vi "Get Element Write Position.vi"(8 "error in (no error)":errorcluster, 11 "CIPC Reference":u64) -> (0 "error out":errorcluster, 3 "Index":u32)   [LabVIEW 2021, in "CIF_NI_CIPC.lvlib"]
doc: "Get element position in the CIPC buffer to which the next element will be written."
uses:
  CIF_NI_CIPC.lvlib
  <vilib>/Utility/error.llb/Trim Whitespace.vi
  <vilib>/Utility/error.llb/Error Cluster From Error Code.vi
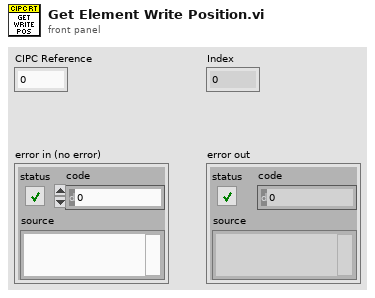
[diagram p1: front panel]
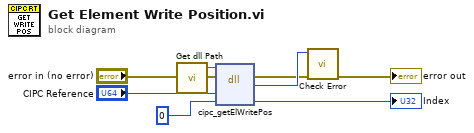
[diagram p0: block diagram]
diagram:
  n1 = call "Get dll Path.vi"() -> ("appended path"=w1:path)  [unwired: 5 in]
  n2 = dll-call lib="libnicipc.*" fn="cipc_getElWritePos"(path in=w1, error in="error in (no error)", "cipc_buffer_ref"="CIPC Reference", "el_index"=u32 0) -> (error out=w5:errorcluster, "return type"=w6:i32, "el_index"=→"Index":u32)  [unwired: 2 in, 1 out]
  n3 = call "Check Error.vi"("error in (no error)"=w5, "Error Code"=w6) -> ("error out"=→"error out":errorcluster)  [unwired: 9 in]
